vi "Update-did-wid-eid.vi"(0 "Device In":T1, 5 "did":string, 7 "wid":string, 9 "eid":string, 11 "error in":errorcluster) -> (4 "Device Out":T1, 15 "error out":errorcluster)   [LabVIEW 2019]
uses:
  _SubVI/Cluster.ctl
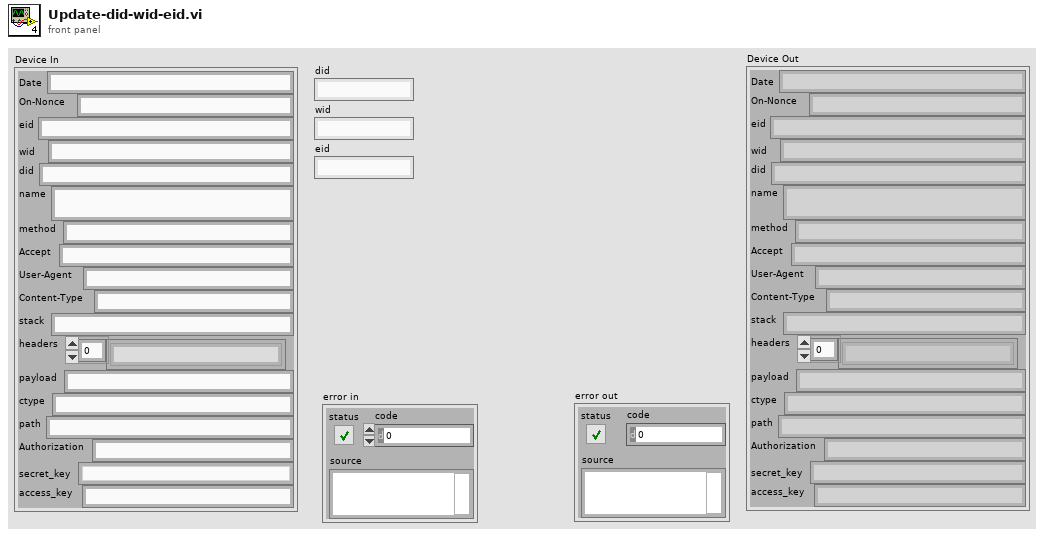
[diagram p1: front panel]
types:
  T1 = typedef "Cluster.ctl" = cluster{"Date":string, "On-Nonce":string, "eid":string, "wid":string, "did":string, "name":string, "method":string, "Accept":string, "User-Agent":string, "Content-Type":string, "stack":string, "headers":string[], "payload":string, "ctype":string, "path":string, "Authorization":string, "secret_key":string, "access_key":string}
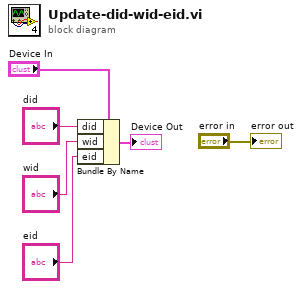
[diagram p0: block diagram]
diagram:
  n1 = Bundle By Name(cluster="Device In", "did"="did", "wid"="wid", "eid"="eid") -> (→"Device Out":T1)
  "error out" <- "error in"
